vi "Get dll Path.vi"() -> (5 "appended path":path)   [LabVIEW 2021, in "CIF_NI_CIPC.lvlib"]
uses:
  CIF_NI_CIPC.lvlib
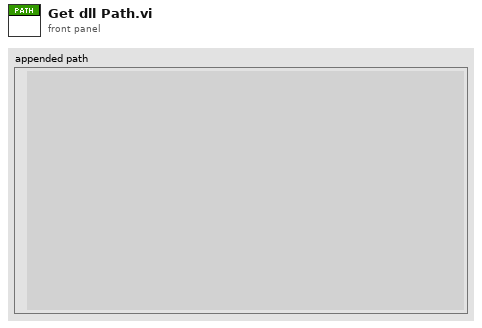
[diagram p1: front panel]
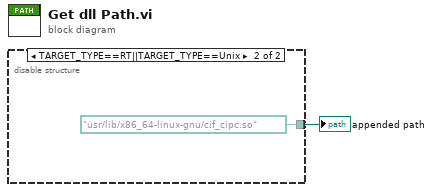
[diagram p0: block diagram]
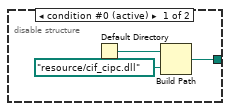
[diagram p2: hidden frame]
diagram:
  n1 = disable-structure shown="TARGET_TYPE==RT||TARGET_TYPE==Unix" {
    disable-tunnel: [w2 path "/usr/lib/x86_64-linux-gnu/cif_cipc.so" ("appended path")] -> w1
    frame condition #0 (active) {
      n2 = Default Directory() -> (w4:path)
      n3 = Build Path(base path=w4, name or relative path=path "resource/cif_cipc.dll") -> (appended path=w2:path)
    }
    frame condition #1 {
    }
  }
  "appended path" <- w1
